vi "DetermineStateOfBoat.vi"() -> (2 "TimeSpentInCurrentState":dbl, 3 "StateOfBoat":T1(ring))   [LabVIEW 2012]
doc: "Eric Schneider and Bonnie Ishiguro\n1/24/14\n\nDetermineStateOfBoat should take in data from the forebrain about the plan of the boat (tacking, jibing, straight, distance to waypoint) as well as robot variables (heading, desired heading, wind speed, etc.) and makes a judgement about the qualitative state of the boat.\n\nThese qualitative states are intended to represent several different rules of sail/rudder control - which rules the sail/rudder should follow should change in each state. The set of current states is by no means set in stone, but should be tweaked with sailing advice so that in the end we have a handful of sailing states that each has a different control scheme for sail/rudder."
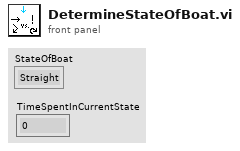
[diagram p1: front panel]
types:
  T1 = enum16{"Straight", "Turning", "Approach Maneuver", "Cross Wind (Tack)", "Cross Wind (Gybe)", "Turtle Mode", ""}
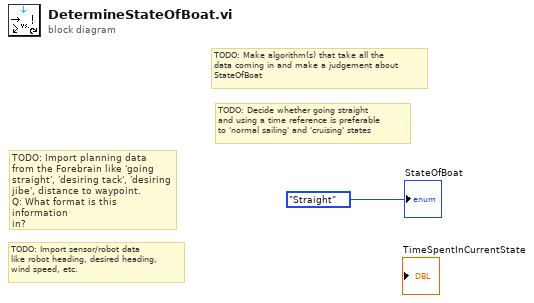
[diagram p0: block diagram]
diagram:
  # "TODO: Decide whether going straight\nand using a time reference is preferable\nto 'normal sailing' and 'cruising' states"
  # "TODO: Make algorithm(s) that take all the\ndata coming in and make a judgement about\nStateOfBoat"
  # "TODO: Import sensor/robot data\nlike robot heading, desired heading,\nwind speed, etc."
  # "TODO: Import planning data\nfrom the Forebrain like 'going\nstraight', 'desiring tack', 'desiring\njibe', distance to waypoint.\nQ: What format is this information\nin?"
  "StateOfBoat" <- T1."Straight"
